vi "2_1.vi"() -> ()   [LabVIEW 2010]
panel:
  out "substring 5":string
  out "substring 4":string
  out "substring 3":string
  out "substring 2":string
  out "substring":string
  out "concatenated string":string
  out "length 5":i32
  out "length 4":i32
  out "length 3":i32
  out "length 2":i32
  out "length":i32
  in  "stop":bool
  in  "OK Button":bool
  in  "String 5":string
  in  "String 4":string
  in  "String 3":string
  in  "String 2":string
  in  "String":string
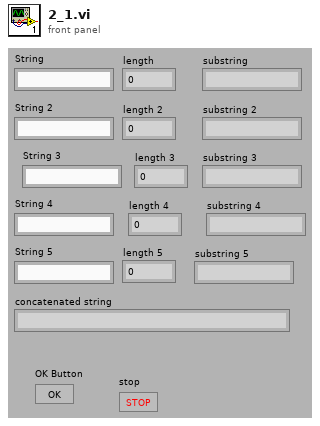
[diagram p1: front panel]
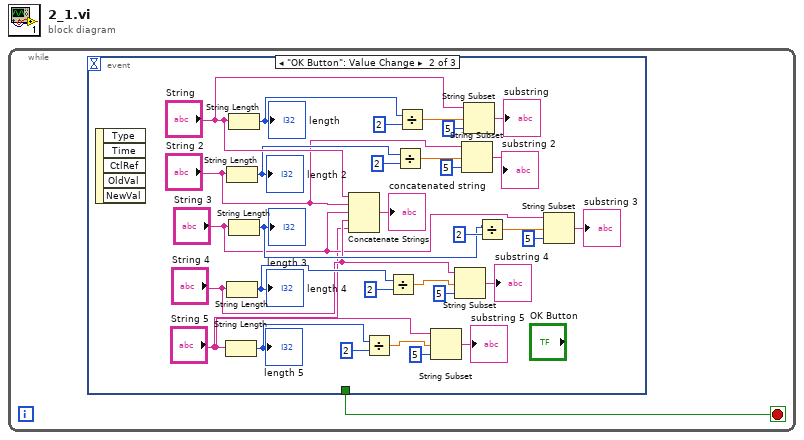
[diagram p0: block diagram]
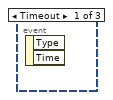
[diagram p2: hidden frame]
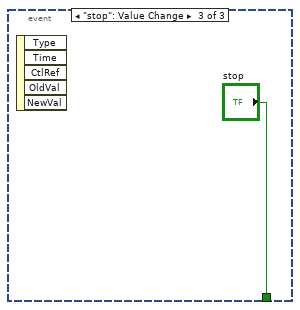
[diagram p3: hidden frame]
diagram:
  n1 = while {
    stop <- w1 stop-if-true
    n2 = event shown="[1] \"OK Button\": Value Change" {
      selector: _ -> [_ _ _]
      dyn-events: _ -> [_ _ _]
      timeout: _ -> [_ _ _]
      tunnel: [_ _ "stop"] -> w1
      event Timeout {
        n3 = event-data() -> ()  [unwired: 1 in, 2 out]
      }
      event "OK Button": Value Change {
        n4 = event-data() -> ()  [unwired: 1 in, 5 out]
        n5 = String Length(string="String 5") -> (length=w8:i32)
        "length 5" <- w8
        n6 = String Length(string="String 2") -> (length=w23:i32)
        "length 2" <- w23
        n7 = String Length(string="String 4") -> (length=w16:i32)
        "length 4" <- w16
        n8 = String Length(string="String") -> (length=w31:i32)
        "length" <- w31
        n9 = String Length(string="String 3") -> (length=w20:i32)
        "length 3" <- w20
        n10 = Concatenate Strings("String", "String 2", "String 3", "String 4", "String 5") -> (→"concatenated string":string)
        n11 = Divide(x=w8, y=2) -> (x/y=w11:dbl)
        n12 = Divide(x=w16, y=2) -> (x/y=w15:dbl)
        n13 = Divide(x=w23, y=2) -> (x/y=w25:dbl)
        n14 = Divide(x=w31, y=2) -> (x/y=w29:dbl)
        n15 = String Subset(string="String 5", offset (0)=w11, length (rest)=5 ("length (rest)")) -> (substring=→"substring 5":string)
        n16 = String Subset(string="String 4", offset (0)=w15, length (rest)=5 ("length (rest)")) -> (substring=→"substring 4":string)
        n17 = String Subset(string="String 2", offset (0)=w25, length (rest)=5 ("length (rest)")) -> (substring=→"substring 2":string)
        n18 = String Subset(string="String", offset (0)=w29, length (rest)=5 ("length (rest)")) -> (substring=→"substring":string)
        n19 = Divide(x=w20, y=2) -> (x/y=w21:dbl)
        n20 = String Subset(string="String 3", offset (0)=w21, length (rest)=5 ("length (rest)")) -> (substring=→"substring 3":string)
      }
      event "stop": Value Change {
        n21 = event-data() -> ()  [unwired: 1 in, 5 out]
      }
    }
  }
